vi "initialisePPData.vi"   [LabVIEW 2013]
uses:
  Controls/postProData.ctl
  Globals/measurementGlobal.vi
types:
  T1 = typedef "postProData.ctl" = cluster{"Channel":string, "Samples":i32, "Mean":dbl, "Standard Deviation":dbl}
  T2 = typedef "chanType.ctl" = enum16{"Default", "Clock", "Pressure Scanner"}
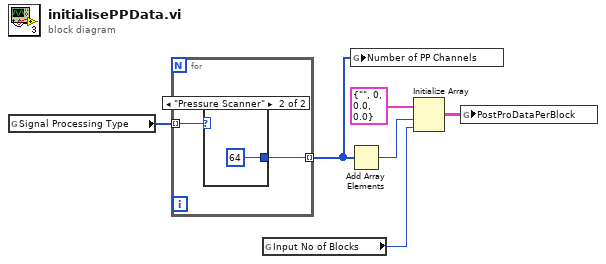
[diagram p0: block diagram]
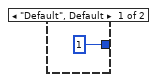
[diagram p2: hidden frame]
diagram:
  n1 = global read "measurementGlobal.vi" "Signal Processing Type"() -> (w6:T2[])
  n2 = for {
    tunnel: w6 -> [w7] mode=indexing
    tunnel: [w8] -> w4 mode=indexing
    n3 = case shown="\"Pressure Scanner\"" w7 {
      tunnel: [1 64] -> w8
      frame "Default", Default {
      }
      frame "Pressure Scanner" {
      }
    }
  }
  n4 = global read "measurementGlobal.vi" "Input No of Blocks"() -> (w5:i32)
  n5 = global write "measurementGlobal.vi" "Number of PP Channels"(w4) -> ()
  n6 = Add Array Elements(numeric array=w4) -> (sum=w3:i32)
  n7 = Initialize Array(T1 {"Channel"="", "Samples"=0, "Mean"=0.0, "Standard Deviation"=0.0} ("Post Pro Data"), w3, w5) -> (w2:T1[][])
  n8 = global write "measurementGlobal.vi" "PostProDataPerBlock"(w2) -> ()
